vi "Read UDP Configuration.vi"(8 "error in (no error)":errorcluster, 11 "Plugin_UI in":refnum<class "Plugin_UI.lvclass">) -> (0 "error out":errorcluster, 2 "Hardware Configuration":T1={"Device Port Number"=2001, "Device IP"="192.168.1.1.100", "Timeout"=5000, "Port Number"=1234}, 3 "Plugin_UI out":refnum<class "Plugin_UI.lvclass">)   [LabVIEW 2020, in "Plugin.lvlib" / "Plugin_UI.lvclass"]
doc: "Read UDP Config"
uses:
  Plugin_UI.lvclass
  UDP Configuration.ctl
  Plugin_UI.lvclass/Plugin_UI.ctl
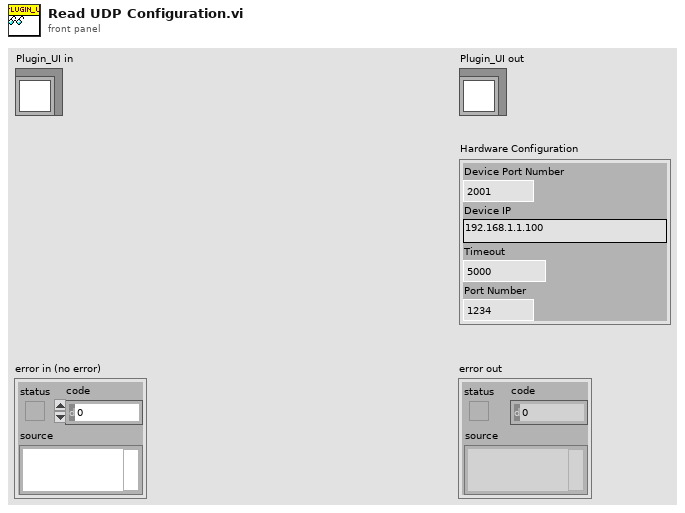
[diagram p1: front panel]
types:
  T1 = typedef "Plugin.lvlib/Plugin_UI.lvclass/UDP Configuration.ctl" = cluster{"Device Port Number":u16, "Device IP":string, "Timeout":i32, "Port Number":u16}
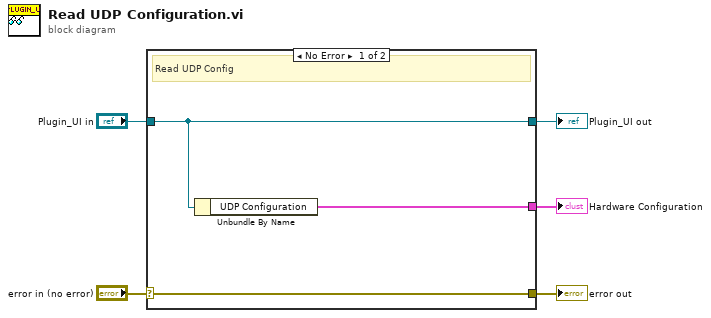
[diagram p0: block diagram]
diagram:
  n1 = case shown="No Error" "error in (no error)" {
    selector: "error in (no error)" -> [w8 w9]
    tunnel: [w8 w9] -> w4
    tunnel: [w7 w10] -> w2
    tunnel: "Plugin_UI in" -> [w7 w10]
    tunnel: [w6 _] -> w1
    frame No Error {
      # "Read UDP Config"
      n2 = Unbundle By Name(w7) -> ("UDP Configuration"=w6:T1)
    }
    frame Error {
    }
  }
  "error out" <- w4
  "Plugin_UI out" <- w2
  "Hardware Configuration" <- w1
